vi "UE9 I2C 24C16A EEPROM.vi"() -> ()   [LabVIEW 2021]
panel:
  out "Read I2C Add":dbl format="%.2f"
  in  "Write":bool
  out "Write I2C Add":dbl format="%.2f"
  in  "Num to Read":u8=8
  in  "Address to read from":u16
  in  "Address to write to":u16
  out "U8 Array Read":u8[](array[numeric])
  in  "U8 Array Write":u8[](array[numeric])=[170, 240, 170, 240]
  out "Error Message":string
  out "error out":errorcluster
  # "I2C example uses the first found USB device.  Writes and reads bytes from the user\narea (0-63) of the 24C01C EEPROM on the LJTick-DAC, which is plugged into FIO0/FIO1.\n\nTested with UD V2.73 and U3 firmware V1.40."
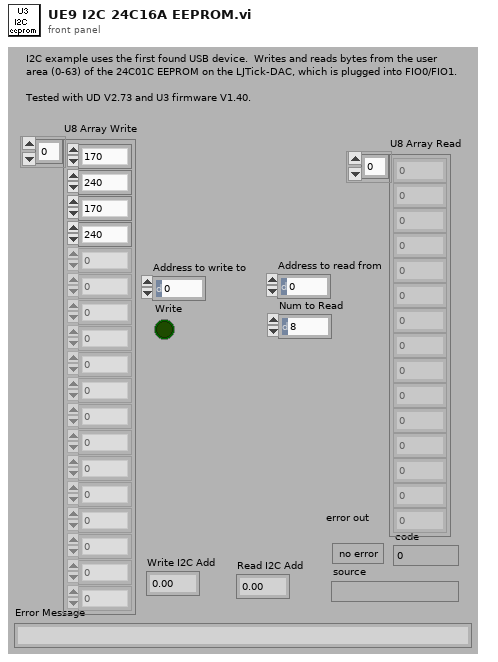
[diagram p1: front panel]
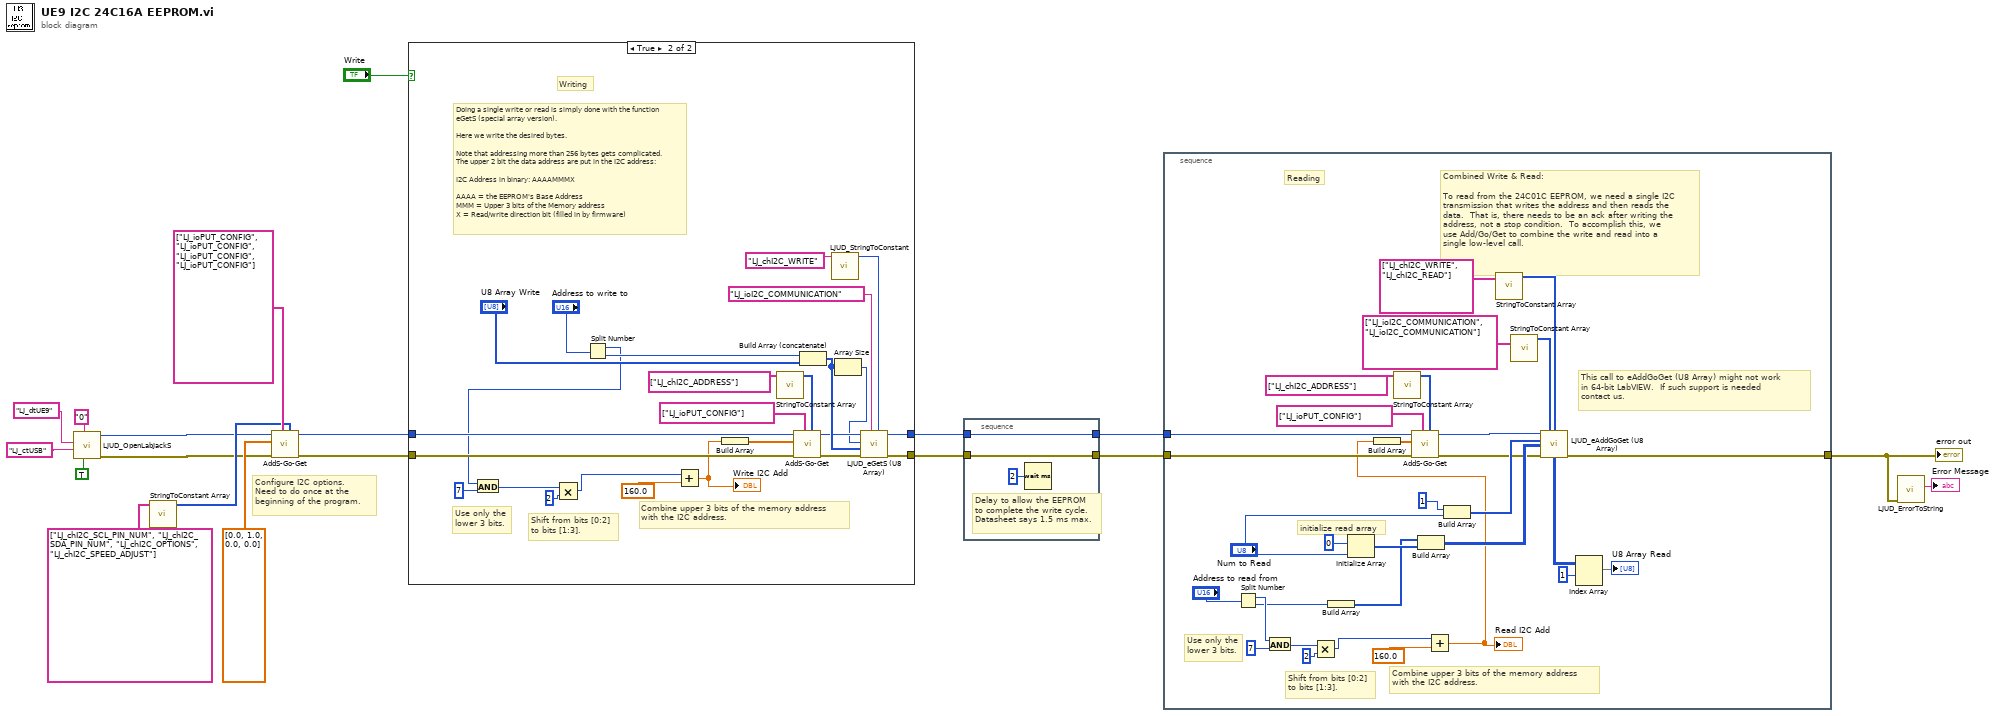
[diagram p0: block diagram]
diagram:
  # "Configure I2C options.\nNeed to do once at the\nbeginning of the program."
  n1 = call "LJUD_OpenLabJackS.vi"("FirstFound"=TRUE, "Address"="0", "ConnectionType"="LJ_ctUSB", "DeviceType"="LJ_dtUE9") -> ("error out"=w10:errorcluster, "Handle"=w9:i32)  [unwired: 5 in, 1 out]
  n2 = call "StringToConstant Array.vi"("String Constant Array In"=string[] ["LJ_chI2C_SCL_PIN_NUM", "LJ_chI2C_SDA_PIN_NUM", "LJ_chI2C_OPTIONS", "LJ_chI2C_SPEED_ADJUST"] ("IOTypes")) -> ("I32 Constant Array Out"=w11:i32[])  [unwired: 10 in]
  n3 = call "AddS-Go-Get.vi"("Channels"=w11, "IOTypes"=string[] ["LJ_ioPUT_CONFIG", "LJ_ioPUT_CONFIG", "LJ_ioPUT_CONFIG", "LJ_ioPUT_CONFIG"], "error in"=w10, "Values Write"=dbl[] [0.0, 1.0, 0.0, 0.0], "Handle In"=w9) -> ("error out"=w3:errorcluster, "Handle Out"=w2:i32)  [unwired: 4 in, 1 out]
  n4 = case shown="True" "Write" {
    tunnel: [w21 w46] -> w7
    tunnel: [w20 w45] -> w5
    tunnel: w3 -> [w21 w44]
    tunnel: w2 -> [w20 w43]
    frame False {
    }
    frame True {
      # "Writing"
      # "Combine upper 3 bits of the memory address\nwith the I2C address."
      # "Shift from bits [0:2]\nto bits [1:3]."
      # "Use only the\nlower 3 bits."
      # "Doing a single write or read is simply done with the function eGetS (special array version).  \n\nHere we write the desired bytes.\n\nNote that addressing more than 256 bytes gets complicated. The upper 2 bit the data address are put in the I2C address:\n\nI2C Address in binary: AAAAMMMX\n\nAAAA = the EEPROM's Base Address\nMMM = Upper 3 bits of the Memory address\nX = Read/write direction bit (filled in by firmware)"
      n5 = Split Number(x="Address to write to") -> (hi(x)=w29:u8, lo(x)=w30:u8)
      n6 = And(x=w29, y=u8 7) -> (x .and. y?=w27:u8)
      n7 = Multiply(x=w27, y=u8 2) -> (x*y=w24:u8)
      n8 = Add(x=w24, y=160.0 ("Value Write")) -> (x+y=w23:dbl)
      "Write I2C Add" <- w23
      n9 = Build Array(w23) -> (w32:dbl[])
      n10 = call "StringToConstant Array.vi"("String Constant Array In"=string[] ["LJ_chI2C_ADDRESS"] ("Array Constant")) -> ("I32 Constant Array Out"=w35:i32[])  [unwired: 10 in]
      n11 = call "AddS-Go-Get.vi"("Channels"=w35, "IOTypes"=string[] ["LJ_ioPUT_CONFIG"] ("Array Constant"), "error in"=w44, "Values Write"=w32, "Handle In"=w43) -> ("error out"=w34:errorcluster, "Handle Out"=w33:i32)  [unwired: 4 in, 1 out]
      n12 = Build Array (concatenate)(w30, "U8 Array Write") -> (w41:u8[])
      n13 = call "LJUD_StringToConstant.vi"("String"="LJ_chI2C_WRITE" ("IOType")) -> ("Constant Number"=w38:i32)  [unwired: 9 in, 1 out]
      n14 = Array Size(array=w41) -> (size(s)=w22:i32)
      n15 = call "LJUD_eGetS (U8 Array).vi"("Channel"=w38, "IOType"="LJ_ioI2C_COMMUNICATION", "error in"=w34, "U8 Array Write"=w41, "Value"=w22, "Handle In"=w33) -> ("error out"=w46:errorcluster, "Handle Out"=w45:i32)  [unwired: 2 in, 2 out]
    }
  }
  n16 = stacked-sequence {
    tunnel: w7 -> [w49]
    tunnel: [w49] -> w6
    tunnel: w5 -> [w48]
    tunnel: [w48] -> w4
    frame #0 {
      # "Delay to allow the EEPROM\nto complete the write cycle.\nDatasheet says 1.5 ms max."
      n17 = Wait (ms)(milliseconds to wait=u32 2) -> ()  [unwired: 1 out]
    }
  }
  n18 = stacked-sequence {
    tunnel: [w81] -> w8
    tunnel: w6 -> [w52]
    tunnel: w4 -> [w51]
    frame #0 {
      # "This call to eAddGoGet (U8 Array) might not work\nin 64-bit LabVIEW.  If such support is needed\ncontact us."
      # "Combine upper 3 bits of the memory address\nwith the I2C address."
      # "Shift from bits [0:2]\nto bits [1:3]."
      # "Use only the\nlower 3 bits."
      # "Reading"
      # "Combined Write & Read:\n\nTo read from the 24C01C EEPROM, we need a single I2C\ntransmission that writes the address and then reads the\ndata.  That is, there needs to be an ack after writing the\naddress, not a stop condition.  To accomplish this, we\nuse Add/Go/Get to combine the write and read into a\nsingle low-level call."
      # "initialize read array"
      n19 = Split Number(x="Address to read from") -> (hi(x)=w61:u8, lo(x)=w60:u8)
      n20 = And(x=w61, y=u8 7) -> (x .and. y?=w66:u8)
      n21 = Multiply(x=w66, y=u8 2) -> (x*y=w63:u8)
      n22 = Build Array(w60) -> (w59:u8[])
      n23 = Initialize Array(u8 0 ("Element Data"), "Num to Read") -> (w73:u8[])
      n24 = call "StringToConstant Array.vi"("String Constant Array In"=string[] ["LJ_chI2C_ADDRESS"] ("Array Constant")) -> ("I32 Constant Array Out"=w56:i32[])  [unwired: 10 in]
      n25 = Build Array(w59, w73) -> (w75:u8[][])
      n26 = Add(x=w63, y=160.0 ("Value Write")) -> (x+y=w50:dbl)
      "Read I2C Add" <- w50
      n27 = Build Array(w50) -> (w55:dbl[])
      n28 = call "AddS-Go-Get.vi"("Channels"=w56, "IOTypes"=string[] ["LJ_ioPUT_CONFIG"] ("Array Constant"), "error in"=w52, "Values Write"=w55, "Handle In"=w51) -> ("error out"=w54:errorcluster, "Handle Out"=w53:i32)  [unwired: 4 in, 1 out]
      n29 = Build Array(1 ("Input Element"), "Num to Read") -> (w78:i32[])
      n30 = call "StringToConstant Array.vi"("String Constant Array In"=string[] ["LJ_chI2C_WRITE", "LJ_chI2C_READ"] ("IOTypes")) -> ("I32 Constant Array Out"=w77:i32[])  [unwired: 10 in]
      n31 = call "StringToConstant Array.vi"("String Constant Array In"=string[] ["LJ_ioI2C_COMMUNICATION", "LJ_ioI2C_COMMUNICATION"] ("IOTypes")) -> ("I32 Constant Array Out"=w76:i32[])  [unwired: 10 in]
      n32 = call "LJUD_eAddGoGet (U8 Array).vi"("Handle In"=w53, "aIOTypes"=w76, "aChannels"=w77, "Values Write"=w78, "ax1s Write (U8 Arrays)"=w75, "error in"=w54) -> ("ax1s Read (U8 Arrays)"=w72:u8[][], "error out"=w81:errorcluster)  [unwired: 3 in, 5 out]
      n33 = Index Array(array=w72, index (row)=1 ("Index (row)")) -> (element=→"U8 Array Read":u8[])  [unwired: 1 in]
    }
  }
  "error out" <- w8
  n34 = call "LJUD_ErrorToString.vi"("error in"=w8) -> ("String"=→"Error Message":string)  [unwired: 10 in]
